vi "Set Sampling Rate.vi"(8 "error in (no error)":errorcluster, 9 "Sampling Rate (Hz) (Default: 1Hz)":T1(ring), 11 "EPU452 in":refnum<class "EPU452.lvclass">) -> (0 "error out":errorcluster, 2 "Response":string, 3 "EPU452 out":refnum<class "EPU452.lvclass">)   [LabVIEW 2018, in "EPU452.lvclass"]
uses:
  EPU452.lvclass
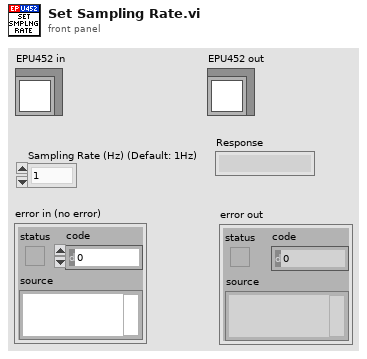
[diagram p1: front panel]
types:
  T1 = enum16{"1", "2", "4", "5", "8", "10", "20", "25", "40", "50", "100"}
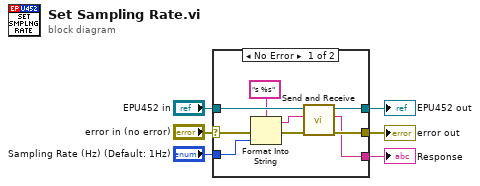
[diagram p0: block diagram]
diagram:
  n1 = case shown="No Error" "error in (no error)" {
    selector: "error in (no error)" -> [w12 w17]
    tunnel: [w10 w17] -> w5
    tunnel: [w9 w16] -> w3
    tunnel: "EPU452 in" -> [w15 w16]
    tunnel: "Sampling Rate (Hz) (Default: 1Hz)" -> [w8 _]
    tunnel: [w7 _] -> w1
    frame No Error {
      n2 = Format Into String(format string="s %s", error in=w12, w8) -> (resulting string=w13:string, error out=w14:errorcluster)  [unwired: 1 in]
      n3 = call "Send and Receive.vi"("error in (no error)"=w14, "Command"=w13, "EPU452 in"=w15) -> ("error out"=w10:errorcluster, "Response"=w7:string, "EPU452 out"=w9:refnum<class "EPU452.lvclass">)  [unwired: 6 in]
    }
    frame Error {
    }
  }
  "error out" <- w5
  "EPU452 out" <- w3
  "Response" <- w1
